vi "v6.vi"() -> ()   [LabVIEW 2023]
uses:
  states_typedef.ctl
panel:
  out "Numeric":i32
  out "Kusur":bool
  out "Kola":bool
  out "Trenutno stanje":T1
  out "Stanje":dbl
  in  "10D":bool
  in  "5D":bool
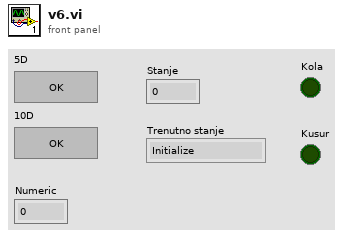
[diagram p1: front panel]
types:
  T1 = typedef "states_typedef.ctl" = enum16{"Initialize", "Wait", "+5D", "+10D", "Izbaci kolu", "Kusur", "Shutdown"}
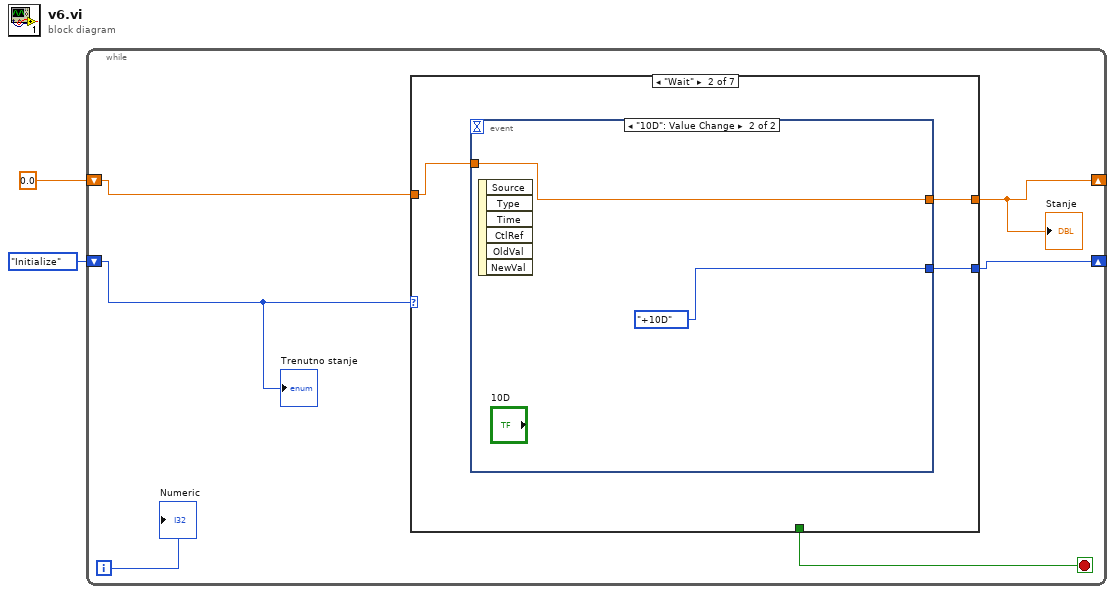
[diagram p0: block diagram]
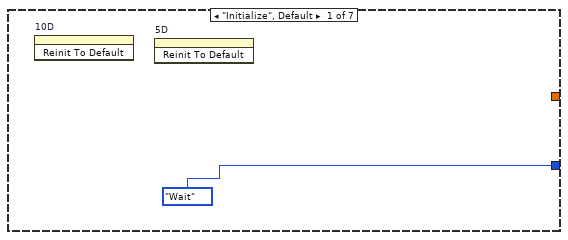
[diagram p2: hidden frame]
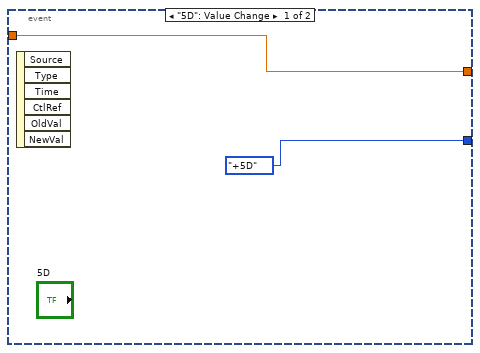
[diagram p3: hidden frame]
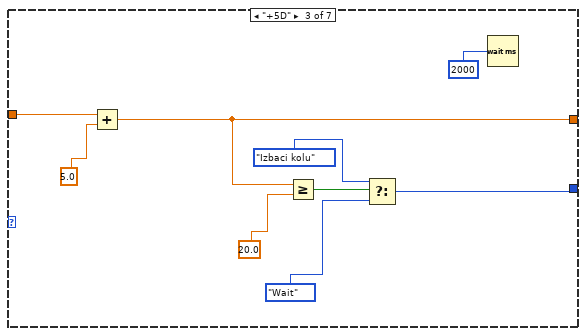
[diagram p4: hidden frame]
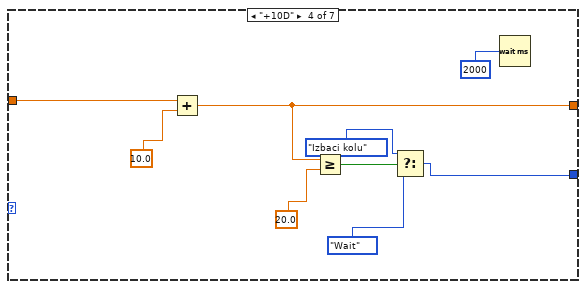
[diagram p5: hidden frame]
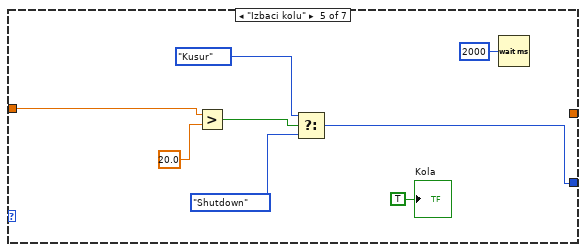
[diagram p6: hidden frame]
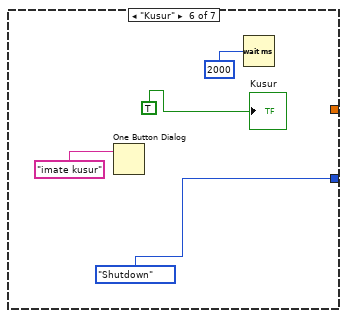
[diagram p7: hidden frame]
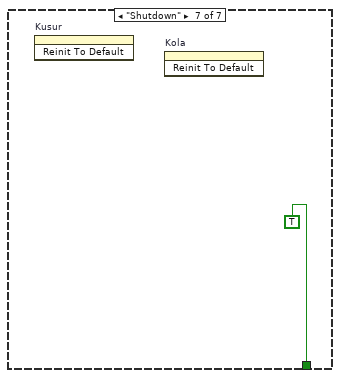
[diagram p8: hidden frame]
diagram:
  n1 = while {
    shift-right: [w4] -> _
    shift-left: states_typedef."Initialize" ("Enum") -> [w6]
    shift-right: [w5] -> _
    shift-left: 0.0 -> [w8]
    i -> [w3]
    stop <- w7 stop-if-true
    n2 = case shown="\"Wait\"" w6 {
      tunnel: [states_typedef."Wait" ("Enum") w12 w18 w27 w39 states_typedef."Shutdown" ("Enum") _] -> w4
      tunnel: w8 -> [_ w11 w24 w34 w38 _ _]
      tunnel: [_ w10 w21 w31 _ _ _] -> w5
      tunnel: [_ _ _ _ _ _ TRUE] -> w7
      frame "Initialize", Default {
        n3 = invoke on="10D" class="Bool" method="Reinit To Default"() -> ()  [unwired: 3 in, 3 out]
        n4 = invoke on="5D" class="Bool" method="Reinit To Default"() -> ()  [unwired: 3 in, 3 out]
      }
      frame "Wait" {
        n5 = event shown="[1] \"10D\": Value Change" {
          selector: _ -> [_ _]
          dyn-events: _ -> [_ _]
          timeout: _ -> [_ _]
          tunnel: [states_typedef."+5D" ("Enum") states_typedef."+10D" ("Enum")] -> w12
          tunnel: w11 -> [w13 w16]
          tunnel: [w13 w16] -> w10
          event "5D": Value Change {
            n6 = event-data() -> ()  [unwired: 1 in, 6 out]
          }
          event "10D": Value Change {
            n7 = event-data() -> ()  [unwired: 1 in, 6 out]
          }
        }
      }
      frame "+5D" {
        n8 = Add(x=w24, y=5.0) -> (x+y=w21:dbl)
        n9 = Greater Or Equal?(x=w21, y=20.0) -> (x >= y?=w23:bool)
        n10 = Select(t=states_typedef."Izbaci kolu" ("Enum"), s=w23, f=states_typedef."Wait" ("Enum")) -> (s? t:f=w18:T1)
        n11 = Wait (ms)(milliseconds to wait=u32 2000) -> ()  [unwired: 1 out]
      }
      frame "+10D" {
        n12 = Add(x=w34, y=10.0) -> (x+y=w31:dbl)
        n13 = Greater Or Equal?(x=w31, y=20.0) -> (x >= y?=w30:bool)
        n14 = Select(t=states_typedef."Izbaci kolu" ("Enum"), s=w30, f=states_typedef."Wait") -> (s? t:f=w27:T1)
        n15 = Wait (ms)(milliseconds to wait=u32 2000) -> ()  [unwired: 1 out]
      }
      frame "Izbaci kolu" {
        n16 = Greater?(x=w38, y=20.0) -> (0:w36:bool)
        n17 = Select(t=states_typedef."Kusur" ("Enum"), s=w36, f=states_typedef."Shutdown") -> (s? t:f=w39:T1)
        n18 = Wait (ms)(milliseconds to wait=u32 2000) -> ()  [unwired: 1 out]
        "Kola" <- TRUE ("Kola")
      }
      frame "Kusur" {
        n19 = One Button Dialog(message="imate kusur") -> ()  [unwired: 1 in, 1 out]
        n20 = Wait (ms)(milliseconds to wait=u32 2000) -> ()  [unwired: 1 out]
        "Kusur" <- TRUE ("Kusur")
      }
      frame "Shutdown" {
        n21 = invoke on="Kusur" class="Bool (strict)" method="Reinit To Default"() -> ()  [unwired: 3 in, 3 out]
        n22 = invoke on="Kola" class="Bool (strict)" method="Reinit To Default"() -> ()  [unwired: 3 in, 3 out]
      }
    }
    "Stanje" <- w5
    "Trenutno stanje" <- w6
    "Numeric" <- w3
  }
